vi "[NameData] - String Array from Cluster or Enum.vi"(8 "Error":errorcluster, 11 "Enum or\nCluster":variant) -> (0 "Error Out":errorcluster, 3 "Data Array Out":string[](array[string]), 5 "Container name":string)   [LabVIEW 2016]
uses:
  <vilib>/Utility/VariantDataType/Type.ctl
  <vilib>/Utility/VariantDataType/VariantType.lvlib
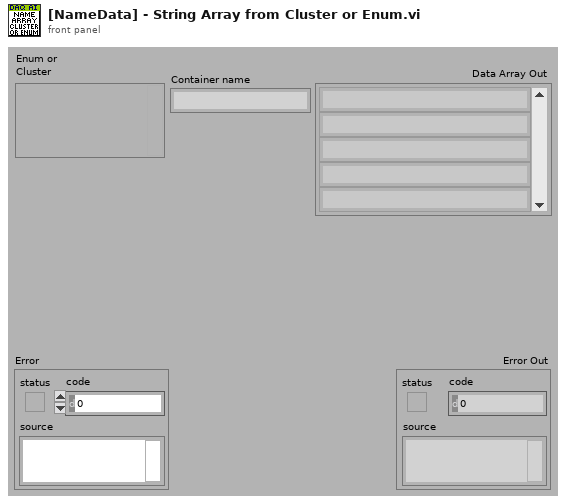
[diagram p1: front panel]
types:
  T1 = typedef "VariantType.lvlib/Type.ctl" = enum8{"Invalid Type", "Void", "I8", "I16", "I32", "I64", "U8", "U16", "U32", "U64", "Single Float", "Double Float", "Extended Float", "Single Complex", "Double Complex", "Extended Complex", "Enum U8", "Enum U16", "Enum U32", "Enum U64", "Single Float With Unit", "Double Float With Unit", "Extended Float With Unit", "Single Complex with Unit", "Double Complex with Unit", "Extended Complex with Unit", "Boolean", "String", "Path", "Picture", "Tag", "Array", "Cluster", "Variant", "LV Variant", "Waveform", "Timestamp", "Digital Waveform", "Digital Data", "ExpressData", "Refnum", "External Data", "VI", "Poly VI", "LabVIEW Class Instance", "Fixed Point"}
  T2 = typedef "VariantType.lvlib/TypedefInfo.ctl" = cluster{"Name":string, "Timestamp":u32}
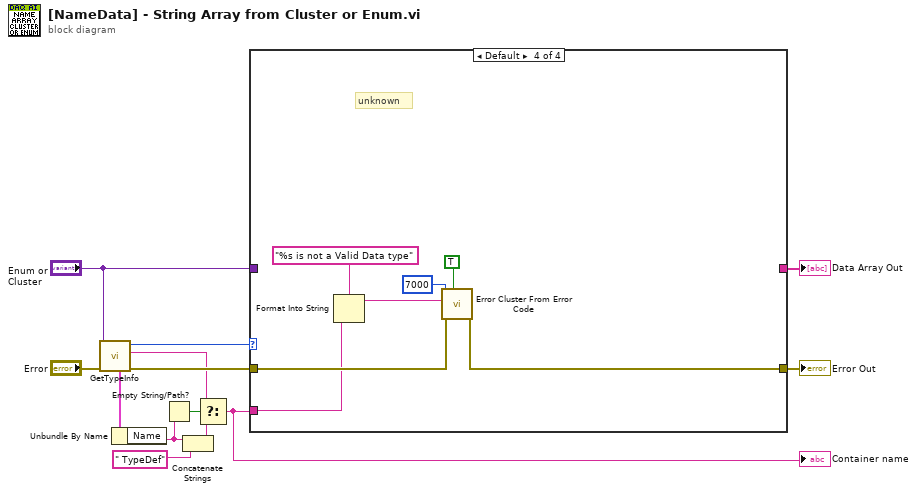
[diagram p0: block diagram]
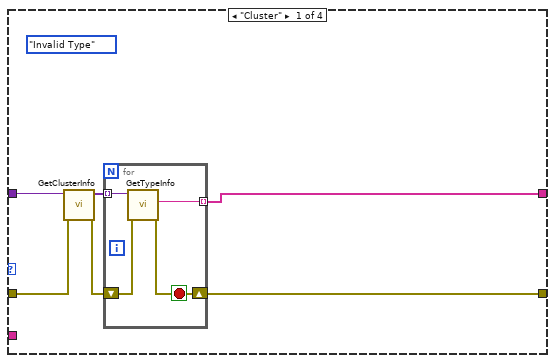
[diagram p2: hidden frame]
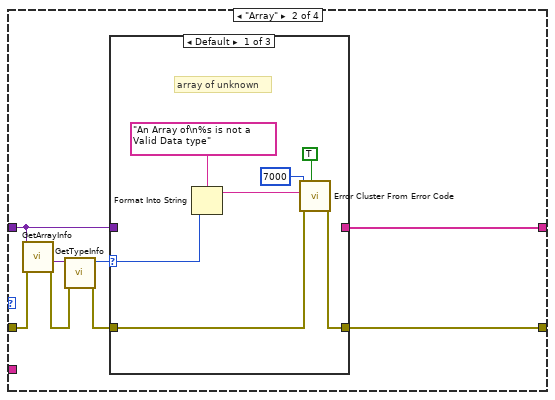
[diagram p3: hidden frame]
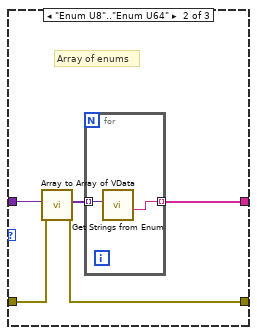
[diagram p4: hidden frame]
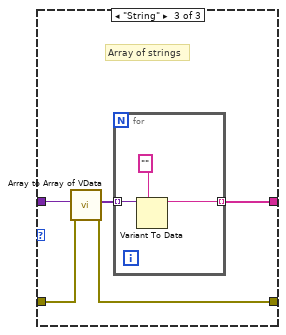
[diagram p5: hidden frame]
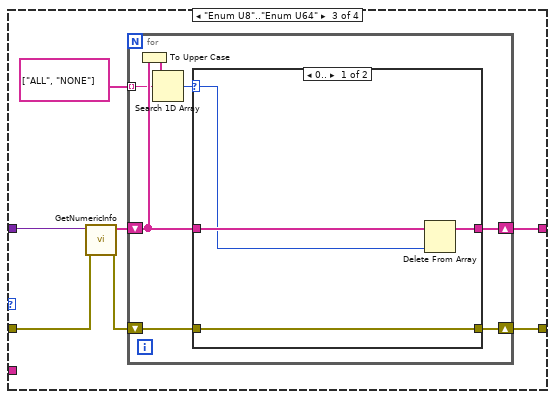
[diagram p6: hidden frame]
diagram:
  n1 = call <vilib>:"GetTypeInfo.vi"("error in (no error)"="Error", "Variant"="Enum or\nCluster") -> ("error out"=w11:errorcluster, "Name"=w8:string, "Type Enum"=w13:T1, "TypedefInfo"=w9:T2)  [unwired: 5 in, 1 out]
  n2 = Unbundle By Name(w9) -> ("Name"=w5:string)
  n3 = Empty String/Path?(string/path=w5) -> (empty?=w6:bool)
  n4 = Concatenate Strings(w5, " TypeDef" ("string")) -> (w4:string)
  n5 = Select(t=w8, s=w6, f=w4) -> (s? t:f=w7:string)
  "Container name" <- w7
  n6 = case shown="Default" w13 {
    tunnel: w11 -> [w18 w30 w59 w76]
    tunnel: "Enum or\nCluster" -> [w19 w31 w60 _]
    tunnel: [w14 w24 w55 _] -> w1
    tunnel: w7 -> [_ _ _ w74]
    tunnel: [w17 w28 w56 w75] -> w2
    frame "Cluster" {
      (unwired) Type."Invalid Type" ("Type Enum")
      n7 = call <vilib>:"GetClusterInfo.vi"("error in (no error)"=w18, "Variant"=w19) -> ("error out"=w16:errorcluster, "Cluster Elements"=w15:variant[])  [unwired: 8 in]
      n8 = for {
        shift-right: [w21] -> w17
        shift-left: w16 -> [w22]
        tunnel: w15 -> [w23] mode=indexing
        tunnel: [w20] -> w14 mode=indexing
        stop <- w21 stop-if-true
        n9 = call <vilib>:"GetTypeInfo.vi"("error in (no error)"=w22, "Variant"=w23) -> ("error out"=w21:errorcluster, "Name"=w20:string)  [unwired: 5 in, 3 out]
      }
    }
    frame "Array" {
      n10 = call <vilib>:"GetArrayInfo.vi"("error in (no error)"=w30, "Variant"=w31) -> ("error out"=w26:errorcluster, "ArrayElement"=w29:variant)  [unwired: 6 in, 2 out]
      n11 = call <vilib>:"GetTypeInfo.vi"("error in (no error)"=w26, "Variant"=w29) -> ("error out"=w25:errorcluster, "Type Enum"=w27:T1)  [unwired: 5 in, 3 out]
      n12 = case shown="Default" w27 {
        selector: w27 -> [w32 _ _]
        tunnel: w31 -> [_ w43 w50]
        tunnel: [w33 w42 w49] -> w28
        tunnel: w25 -> [w34 w41 w48]
        tunnel: [_ w39 w46] -> w24
        frame Default {
          # "array of unknown"
          n13 = Format Into String(format string="An Array of\n%s is not a Valid Data type" ("error message (\"\")"), w32) -> (resulting string=w36:string)  [unwired: 2 in, 1 out]
          n14 = call <vilib>:"Error Cluster From Error Code.vi"("show call chain? (False)"=TRUE, "error in (no error)"=w34, "error message (\"\")"=w36, "error code (0)"=7000) -> ("error out"=w33:errorcluster)  [unwired: 5 in]
        }
        frame "Enum U8".."Enum U64" {
          # "Array of enums"
          n15 = call "Array to Array of VData.vi"("error in (no error)"=w41, "MultiD Array"=w43) -> ("error out"=w42:errorcluster, "1D Array of Variants"=w40:variant[])  [unwired: 8 in]
          n16 = for {
            tunnel: w40 -> [w45] mode=indexing
            tunnel: [w44] -> w39 mode=indexing
            n17 = call "Get Strings from Enum.vi"("Enum"=w45) -> ("String Value"=w44:string)  [unwired: 7 in, 3 out]
          }
        }
        frame "String" {
          # "Array of strings"
          n18 = call "Array to Array of VData.vi"("error in (no error)"=w48, "MultiD Array"=w50) -> ("error out"=w49:errorcluster, "1D Array of Variants"=w47:variant[])  [unwired: 8 in]
          n19 = for {
            tunnel: w47 -> [w53] mode=indexing
            tunnel: [w51] -> w46 mode=indexing
            n20 = Variant To Data(type="" ("String Value"), Variant=w53) -> (data=w51:string)  [unwired: 1 in, 1 out]
          }
        }
      }
    }
    frame "Enum U8".."Enum U64" {
      n21 = call <vilib>:"GetNumericInfo.vi"("error in (no error)"=w59, "Variant"=w60) -> ("error out"=w58:errorcluster, "EnumNames"=w57:string[])  [unwired: 6 in, 2 out]
      n22 = for {
        shift-right: [w62] -> w55
        shift-left: w57 -> [w64]
        tunnel: string[] ["ALL", "NONE"] -> [w61] mode=indexing
        shift-right: [w63] -> w56
        shift-left: w58 -> [w65]
        n23 = To Upper Case(1:w64) -> (0:w67:string[])
        n24 = Search 1D Array(1D array=w67, element=w61) -> (index of element=w66:i32)  [unwired: 1 in]
        n25 = case shown="0.." w66 {
          selector: w66 -> [w69 _]
          tunnel: w65 -> [w71 w73]
          tunnel: [w71 w73] -> w63
          tunnel: w64 -> [w70 w72]
          tunnel: [w68 w72] -> w62
          frame 0.. {
            n26 = Delete From Array(array=w70, index=w69) -> (array with subset deleted=w68:string[])  [unwired: 1 in, 1 out]
          }
          frame ..-1 {
          }
        }
      }
    }
    frame Default {
      # "unknown"
      n27 = Format Into String(format string="%s is not a Valid Data type" ("error message (\"\")"), w74) -> (resulting string=w79:string)  [unwired: 2 in, 1 out]
      n28 = call <vilib>:"Error Cluster From Error Code.vi"("show call chain? (False)"=TRUE, "error in (no error)"=w76, "error message (\"\")"=w79, "error code (0)"=7000) -> ("error out"=w75:errorcluster)  [unwired: 5 in]
    }
  }
  "Data Array Out" <- w1
  "Error Out" <- w2
